vi "SDF Small Gasifier HMI - Main.vi"() -> (0 "error out":errorcluster)   [LabVIEW 2013]
doc: "This VI is responsible for the HMI's page navigation. This is where all the pages exist."
uses:
  <vilib>/NI/Current Value Table/Type Defs/Single Tag.ctl
  <vilib>/NI/Current Value Table/Type Defs/Data Types.ctl
  <vilib>/NI/CCC/Tag Configuration.ctl
  <vilib>/NI/CCC/Tag Direction.ctl
  <vilib>/NI/Current Value Table/Type Defs/File Format.ctl
  <vilib>/NI/Current Value Table/Type Defs/Tag Grouping set.ctl
  <vilib>/Utility/file.llb/Read From Spreadsheet File (string).vi
  <vilib>/NI/Current Value Table/Current Value Table.lvlib
  <vilib>/NI/CCC/NI_CCC.lvlib
panel:
  out "Invalid CCC Tags":T1[](array[typedef])
  out "CCC Tags":T1[](array[typedef])
  out "CVT Tags":T4[](array[typedef])
  out "Invalid  CVT Tags":T4[](array[typedef])
  in  "stop":bool
  # "<< Update to match your controller IP address"
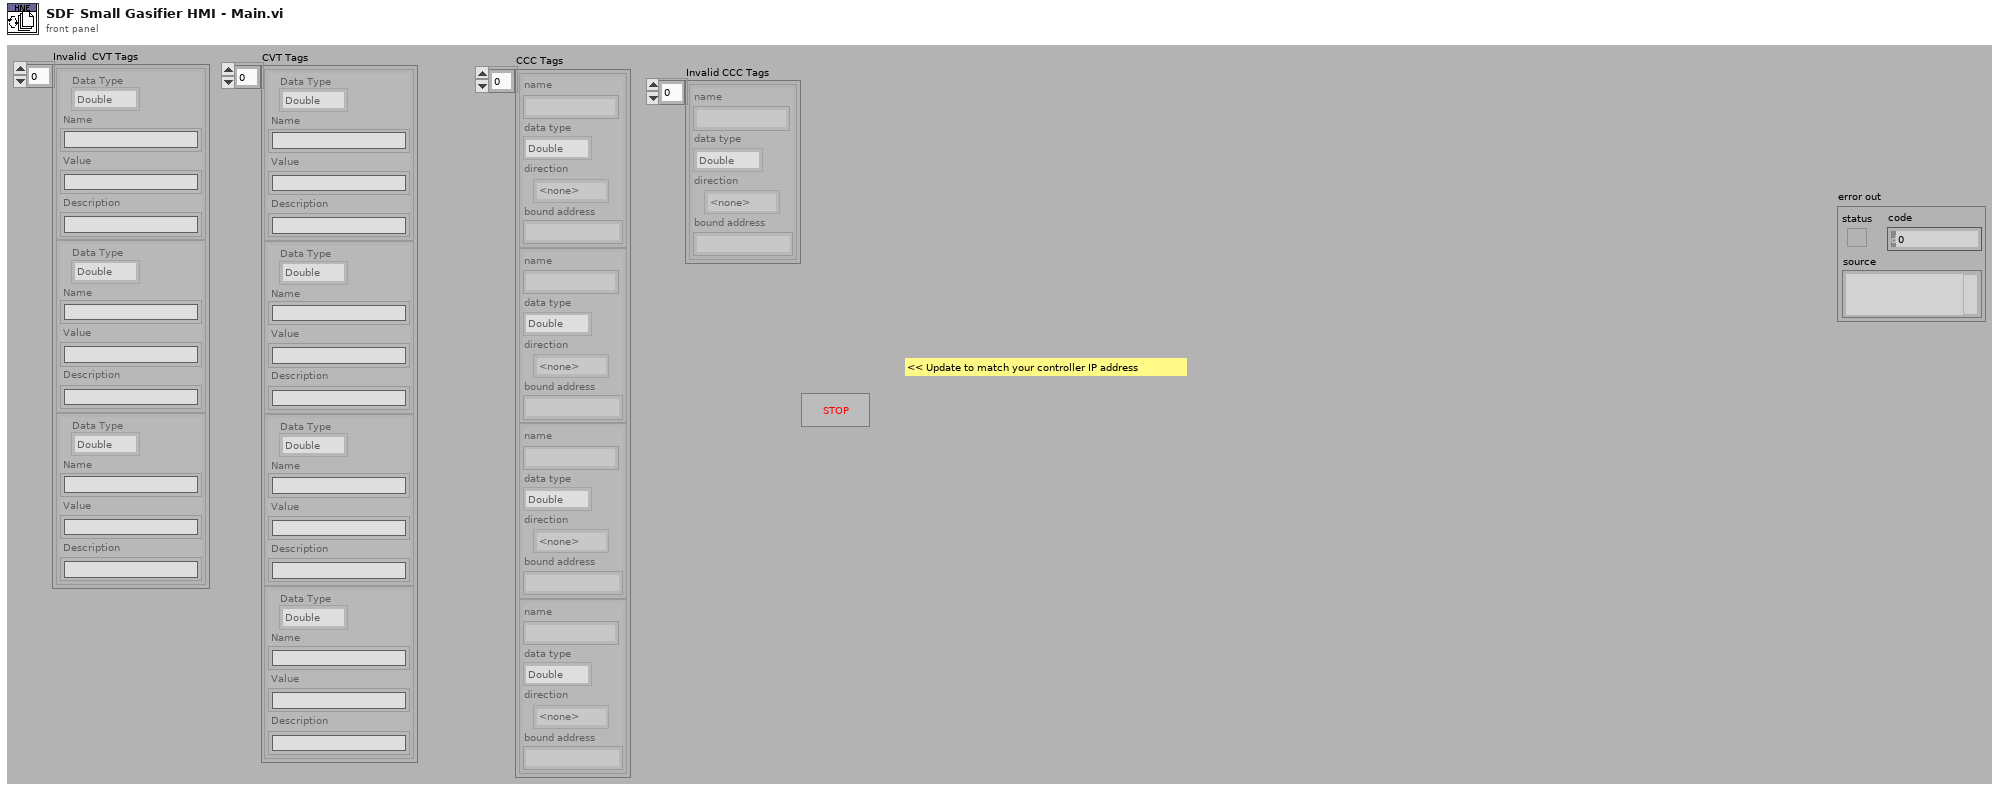
[diagram p1: front panel]
types:
  T1 = typedef "NI_CCC.lvlib/Tag Configuration.ctl" = cluster{"name":string, "data type":T2, "direction":T3, "bound address":string}
  T2 = typedef "Current Value Table.lvlib/Data Types.ctl" = enum16{"Double", "Single", "I64", "I32", "I16", "I8", "U64", "U32", "U16", "U8", "String", "Boolean", "Array of U8", "Array of U16", "Array of U32", "Array of U64", "Array of I64", "Array of I32", "Array of I16", "Array of I8", "Array of Double", "Array of Single", "Array of Boolean", "Array of String"}
  T3 = typedef "NI_CCC.lvlib/Tag Direction.ctl" = enum32{"<none>", "Read", "Write"}
  T4 = typedef "Current Value Table.lvlib/Single Tag.ctl" = cluster{"Data Type":T2, "Name":string, "Value":string, "Description":string}
  T5 = typedef "Current Value Table.lvlib/File Format.ctl" = cluster{"Tags":T4[], "Group Listings":T6[]}
  T6 = typedef "Current Value Table.lvlib/Tag Grouping set.ctl" = cluster{"Group":string, "Tag Names":string[]}
  T7 = typedef "NI_CCC.lvlib/Connection ID.ctl" = cluster{"server ID":string, "connection ID":T8, "meta data":T9[], "write tag list":T1[], "read tag list":T1[]}
  T8 = typedef "NI STM.lvlib/TCP Connection Info.ctl" = cluster{"connection ID":refnum<k5>, "meta data":T9[]}
  T9 = typedef "NI STM.lvlib/MetaDataElement.ctl" = string
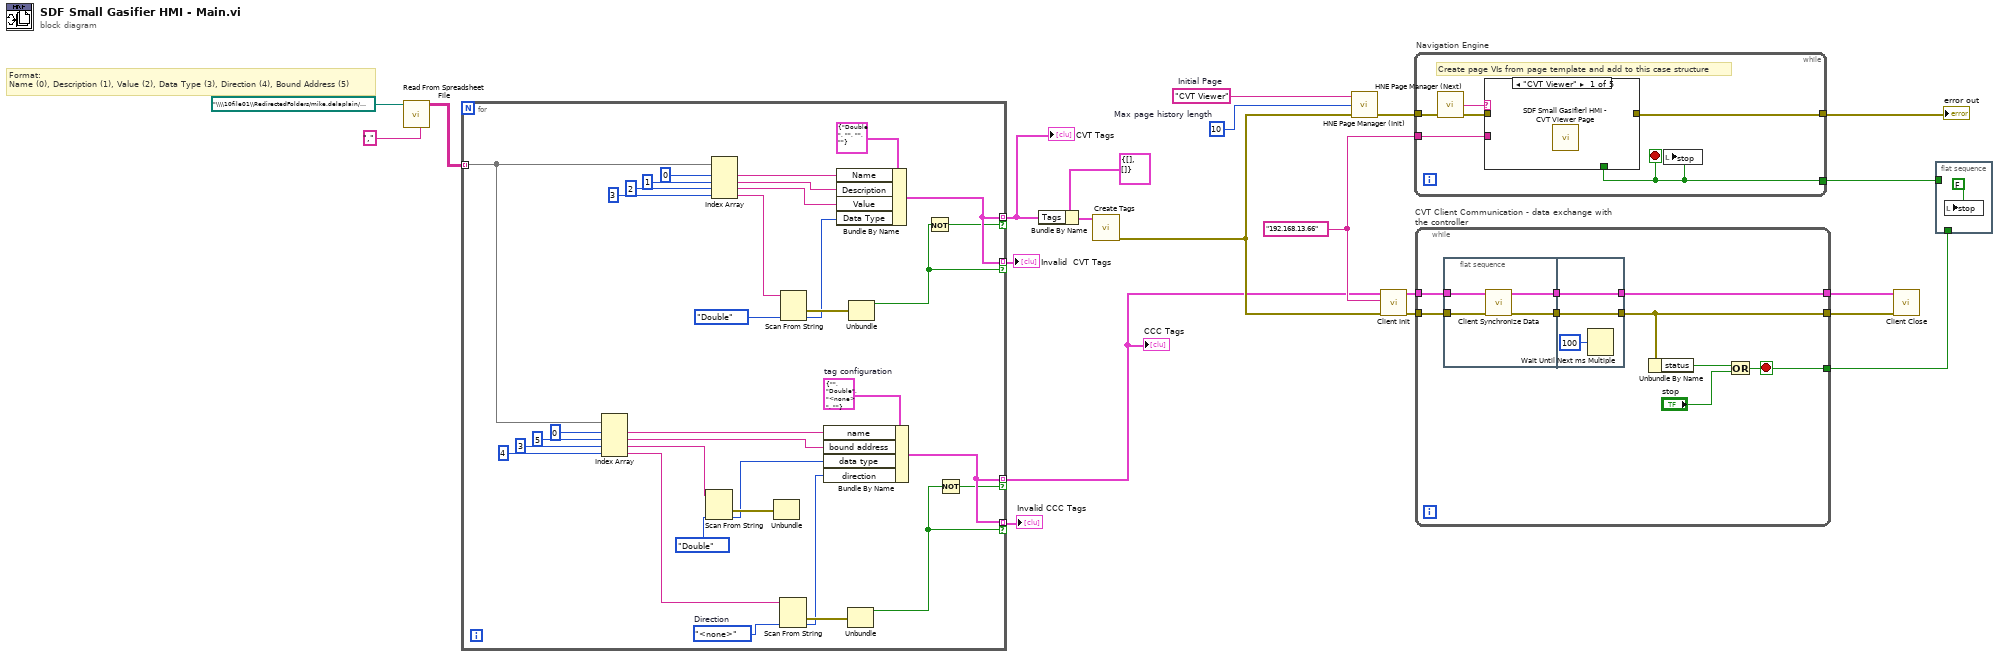
[diagram p0: block diagram]
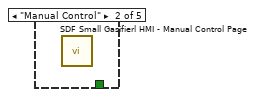
[diagram p2: hidden frame]
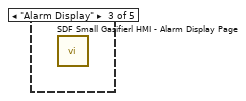
[diagram p3: hidden frame]
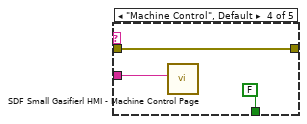
[diagram p4: hidden frame]
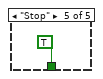
[diagram p5: hidden frame]
diagram:
  w6 = "192.168.13.66" ("Target IP Address")
  w21 = 10  # Max page history length
  w20 = "CVT Viewer"  # Initial Page
  # "Format:\nName (0), Description (1), Value (2), Data Type (3), Direction (4), Bound Address (5)"
  n1 = call-poly <vilib>:"Read From Spreadsheet File.vi"("delimiter (\\t)"="," ("delimiter (\\t)"), "file path (dialog if empty)"=path "\\\\10file01\\RedirectedFolders/mike.delaplain/Documents/LabVIEW/SDF Small Gasifier/Tags.csv") -> ("all rows"=w15:string[][])  [unwired: 5 in, 4 out]
  n2 = for {
    tunnel: w15 -> [w33] mode=indexing
    tunnel: [w52] -> w12 mode=indexing if=w50
    tunnel: [w52] -> w10 mode=indexing if=w51
    tunnel: [w24] -> w2 mode=indexing if=w23
    tunnel: [w24] -> w1 mode=indexing if=w22
    w25 = Tag_Direction."<none>"  # Direction
    w32 = T1 {"name"="", "data type"=enum."Double", "direction"=enum."<none>", "bound address"=""}  # tag configuration
    n3 = Index Array(array=w33, index #1=0 ("index"), index #2=5 ("index"), index #3=3 ("index"), index #4=4 ("index")) -> (element #1=w40:string, element #2=w34:string, element #3=w29:string, element #4=w27:string)
    n4 = Scan From String(input string=w29, default 1=Data_Types."Double" ("Data Type")) -> (error out=w30:errorcluster, output 1=w28:T2)  [unwired: 3 in, 2 out]
    n5 = Index Array(array=w33, index #1=0 ("index"), index #2=1 ("index"), index #3=2 ("index"), index #4=3 ("index")) -> (element #1=w54:string, element #2=w44:string, element #3=w43:string, element #4=w42:string)
    n6 = Unbundle(w30) -> ()  [unwired: 3 out]
    n7 = Scan From String(input string=w27, default 1=w25) -> (error out=w39:errorcluster, output 1=w26:T3)  [unwired: 3 in, 2 out]
    n8 = Scan From String(input string=w42, default 1=Data_Types."Double" ("Data Type")) -> (error out=w53:errorcluster, output 1=w41:T2)  [unwired: 3 in, 2 out]
    n9 = Bundle By Name(cluster=w32, "name"=w40, "bound address"=w34, "data type"=w28, "direction"=w26) -> (w24:T1)
    n10 = Bundle By Name(cluster=T4 {"Data Type"=enum."Double", "Name"="", "Value"="", "Description"=""} ("Tag"), "Name"=w54, "Description"=w44, "Value"=w43, "Data Type"=w41) -> (w52:T4)
    n11 = Unbundle(w39) -> ("status"=w22:bool)  [unwired: 2 out]
    n12 = Unbundle(w53) -> ("status"=w50:bool)  [unwired: 2 out]
    n13 = Not(x=w50) -> (.not. x?=w51:bool)
    n14 = Not(x=w22) -> (.not. x?=w23:bool)
  }
  "Invalid  CVT Tags" <- w12
  "CVT Tags" <- w10
  "CCC Tags" <- w2
  "Invalid CCC Tags" <- w1
  n15 = Bundle By Name(cluster=T5 {"Tags"=[], "Group Listings"=[]} ("CVT Tags to Create"), "Tags"=w10) -> (w13:T5)
  n16 = call <vilib>:"Create Tags.vi"("CVT Tags to Create"=w13) -> ("error out"=w3:errorcluster)  [unwired: 10 in]
  n17 = call <userlib>:"HNE Page Manager (Init).vi"("error in (no error)"=w3, "Max page history length"=w21, "Initial Page"=w20) -> ("error out"=w19:errorcluster)  [unwired: 2 in]
  n18 = call <vilib>:"Client Init.vi"("error in"=w3, "server IP address"=w6, "tag list"=w2) -> ("error out"=w4:errorcluster, "connection ID"=w5:T7)  [unwired: 7 in]
  n19 = while "Navigation Engine" {
    tunnel: w19 -> [w60]
    tunnel: [w58] -> w18
    tunnel: [w57] -> w17
    tunnel: w6 -> [w56]
    stop <- w57 stop-if-true
    # "Create page VIs from page template and add to this case structure"
    n20 = call <userlib>:"HNE Page Manager (Next).vi"("error in (no error)"=w60) -> ("error out"=w59:errorcluster, "Next Page"=w61:string)  [unwired: 3 in]
    n21 = case shown="\"CVT Viewer\"" w61 {
      tunnel: [_ _ _ FALSE TRUE] -> w57
      tunnel: w59 -> [_ _ _ w64 _]
      tunnel: [_ _ _ w64 _] -> w58
      tunnel: w56 -> [_ _ _ w63 _]
      frame "CVT Viewer" {
        n22 = call "SDF Small Gasifierl HMI - CVT Viewer Page.vi"() -> ()  [unwired: 12 in]
      }
      frame "Manual Control" {
        n23 = call "SDF Small Gasifierl HMI - Manual Control Page.vi"() -> ()  [unwired: 12 in]
      }
      frame "Alarm Display" {
        n24 = call "SDF Small Gasifierl HMI - Alarm Display Page.vi"() -> ()  [unwired: 12 in]
      }
      frame "Machine Control", Default {
        n25 = call "SDF Small Gasifierl HMI - Machine Control Page.vi"("Receiver Host"=w63) -> ()  [unwired: 11 in]
      }
      frame "Stop" {
      }
    }
    n26 = local write "stop"(w57) -> ()
  }
  "error out" <- w18
  n27 = while "CVT Client Communication - data exchange with the controller" {
    tunnel: w5 -> [w74]
    tunnel: w4 -> [w73]
    tunnel: [w71] -> w7
    tunnel: [w69] -> w8
    tunnel: [w68] -> w16
    stop <- w68 stop-if-true
    n28 = flat-sequence {
      tunnel: [w77] -> w72
      tunnel: [w75] -> w70
      tunnel: w74 -> [w78]
      tunnel: w73 -> [w76]
      tunnel: [w80] -> w71
      tunnel: w72 -> [w80]
      tunnel: [w79] -> w69
      tunnel: w70 -> [w79]
      frame #0 {
        n29 = call <vilib>:"Client Synchronize Data.vi"("error in"=w76, "connection ID in"=w78) -> ("error out"=w75:errorcluster, "connection ID out"=w77:T7)  [unwired: 8 in]
      }
      frame #1 {
        n30 = Wait Until Next ms Multiple(millisecond multiple=u32 100) -> ()  [unwired: 1 out]
      }
    }
    n31 = Unbundle By Name(w69) -> ("status"=w67:bool)
    n32 = Or(x=w67, y="stop") -> (x .or. y?=w68:bool)
  }
  n33 = call <vilib>:"Client Close.vi"("error in"=w8, "connection ID"=w7) -> ()  [unwired: 9 in, 1 out]
  n34 = flat-sequence {
    tunnel: w17 -> [_]
    tunnel: w16 -> [_]
    frame #0 {
      n35 = local write "stop"(FALSE) -> ()
    }
  }
